vi "RC_Client.vi"(8 "error in (no error)":errorcluster, 10 "ID":i32, 11 "RemoteControl in":refnum<class "RemoteControl.lvclass">) -> (0 "error out":errorcluster)   [LabVIEW 2019, in "RemoteControl.lvlib" / "RemoteControl.lvclass"]
uses:
  RemoteControl.lvclass
  <userlib>/_OpenG.lib/error/error.llb/Filter Error Codes (Array)__ogtk.vi
  b7e1e2dc-a0d6-4bbd-afea-6de24c297ea6.vi
panel:
  in  "milliseconds to wait":u32
  out "time (1 message) (s)":dbl
  out "startup time (s)":dbl
  out "messages/s":dbl
  in  "remote port":u16=6341
  in  "address":string
  out "Response":string
  out "Messages":i32
  in  "Stop":bool
  out "Command reponse":string
  out "Command":string
  out "meta data\n(available commands)":string
  # "CLIENT (API)"
  # "Connection info"
  # "Message Sent"
  # "Message Received"
  # "Metrics"
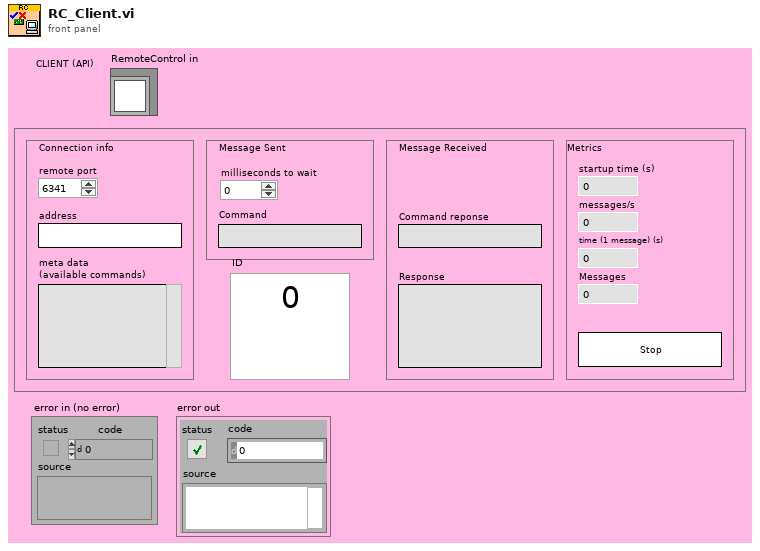
[diagram p1: front panel]
types:
  T1 = cluster{"Command out":string, "Data out":variant, string}
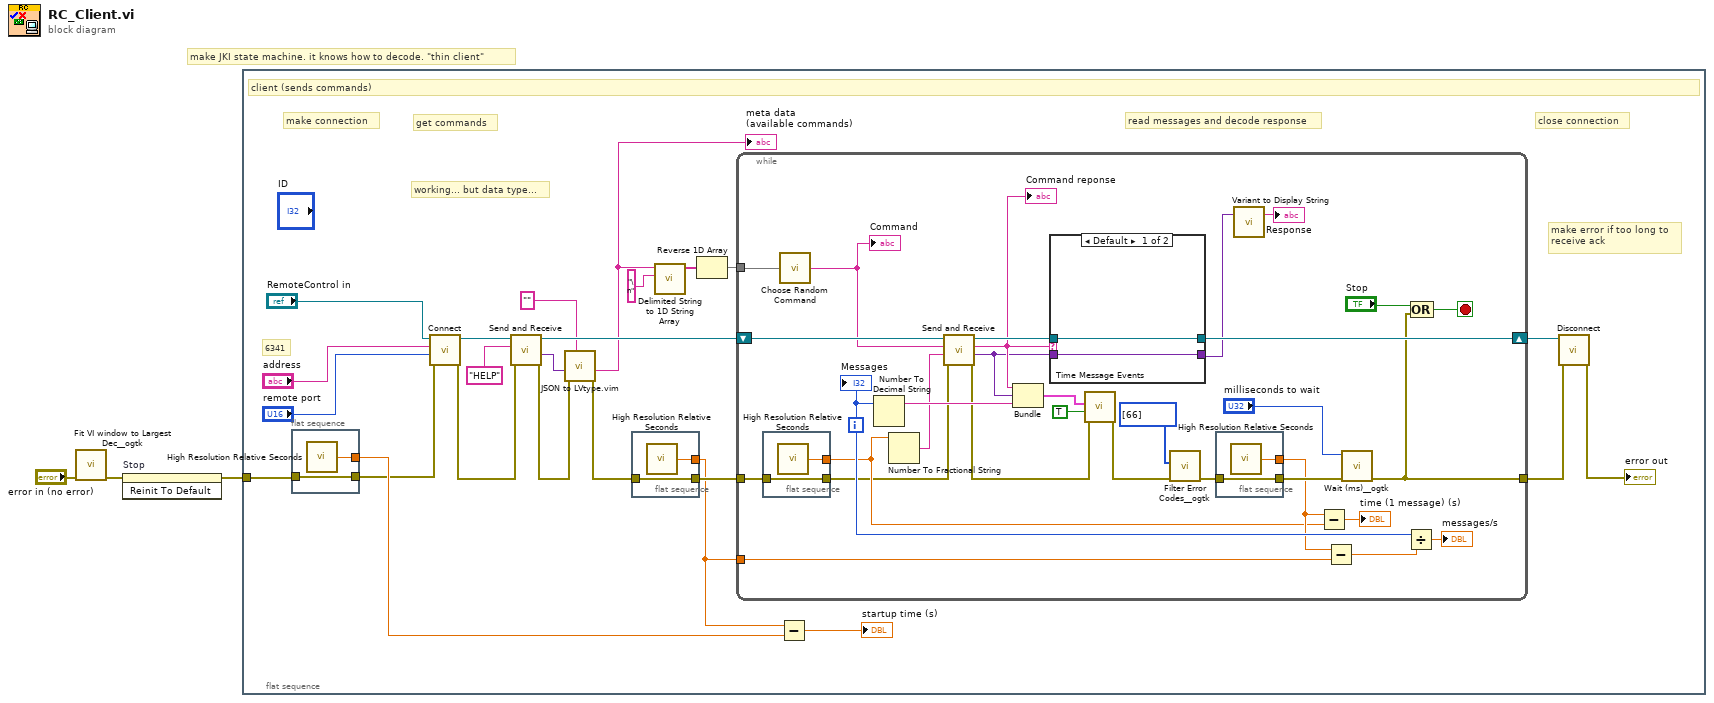
[diagram p0: block diagram]
diagram:
  # "make JKI state machine. it knows how to decode. \"thin client\""
  n1 = call <userlib>:"Fit VI window to Largest Dec__ogtk.vi"("error in (no error)"="error in (no error)") -> ("error out"=w3:errorcluster)  [unwired: 5 in, 1 out]
  n2 = invoke on="Stop" class="Bool" method="Reinit To Default"(error in=w3) -> (error out=w2:errorcluster)  [unwired: 2 in, 2 out]
  n3 = flat-sequence {
    tunnel: w2 -> [w23]
    frame #0 {
      # "working... but data type..."
      # "close connection"
      # "read messages and decode response"
      # "get commands"
      # "make connection"
      # "6341"
      # "make error if too long to\nreceive ack"
      # "client (sends commands)"
      n4 = flat-sequence {
        tunnel: [w28] -> w16
        tunnel: [w29] -> w22
        tunnel: w23 -> [w28]
        frame #0 {
          n5 = call <vilib>:"High Resolution Relative Seconds.vi"() -> ("relative seconds"=w29:dbl)
        }
      }
      n6 = call "Connect.vi"("error in (no error)"=w16, "Port"="remote port", "address"="address", "RemoteControl in"="RemoteControl in") -> ("error out"=w10:errorcluster, "RemoteControl out"=w11:refnum<class "RemoteControl.lvclass">)  [unwired: 6 in]
      n7 = call "Send and Receive.vi"("error in (no error)"=w10, "Command"="HELP", "RemoteControl in"=w11) -> ("error out"=w5:errorcluster, "Data out"=w8:variant, "RemoteControl out"=w9:refnum<class "RemoteControl.lvclass">)  [unwired: 5 in, 1 out]
      n8 = call "JSON to LVtype.vim"("type"="", "error in (no error)"=w5, "JSON Data in"=w8) -> ("error out"=w4:errorcluster, "Data out"=w6:string)  [unwired: 7 in]
      "meta data\n(available commands)" <- w6
      n9 = flat-sequence {
        tunnel: [w30] -> w26
        tunnel: [w31] -> w24
        tunnel: w4 -> [w30]
        frame #0 {
          n10 = call <vilib>:"High Resolution Relative Seconds.vi"() -> ("relative seconds"=w31:dbl)
        }
      }
      n11 = call <vilib>:"Delimited String to 1D String Array.vi"("delimiter"="\n", "delimited string"=w6) -> ("string array"=w21:string[])  [unwired: 9 in]
      n12 = Reverse 1D Array(array=w21) -> (reversed array=w27:string[])
      n13 = while {
        tunnel: [w54] -> w14
        tunnel: w26 -> [w47]
        tunnel: w27 -> [w46]
        tunnel: w24 -> [w57]
        shift-right: [w55] -> w15
        shift-left: w9 -> [w41]
        i -> [w53]
        stop <- w52 stop-if-true
        n14 = flat-sequence {
          tunnel: [w63] -> w38
          tunnel: [w64] -> w44
          tunnel: w47 -> [w63]
          frame #0 {
            n15 = call <vilib>:"High Resolution Relative Seconds.vi"() -> ("relative seconds"=w64:dbl)
          }
        }
        n16 = call "Choose Random Command.vi"("Array"=w46) -> ("String"=w40:string)
        "Command" <- w40
        n17 = Number To Decimal String(number=w53) -> (decimal integer string=w45:string)  [unwired: 1 in]
        n18 = Number To Fractional String(number=w44) -> (F-format string=w39:string)  [unwired: 3 in]
        n19 = call "Send and Receive.vi"("error in (no error)"=w38, "Data"=w39, "Command"=w40, "RemoteControl in"=w41) -> ("error out"=w37:errorcluster, "Data out"=w34:variant, "Command out"=w35:string, "RemoteControl out"=w36:refnum<class "RemoteControl.lvclass">)  [unwired: 4 in]
        "Command reponse" <- w35
        n20 = Bundle("Command out"=w35, "Data out"=w34, w45) -> (w43:T1)  [unwired: 1 in]
        n21 = case shown="Default" w35 {
          tunnel: [w67 w69] -> w32
          tunnel: w36 -> [w68 w70]
          tunnel: w34 -> [w67 w69]
          tunnel: [w68 w70] -> w55
          frame Default {
          }
          frame "HELP" {
          }
        }
        n22 = call "Time Message Events.vi"("error in (no error)"=w37, "Debug Mode"=TRUE, "Message in"=w43) -> ("error out"=w56:errorcluster)  [unwired: 5 in, 3 out]
        n23 = call-poly <userlib>:"Filter Error Codes__ogtk.vi"("Error In"=w56, "Error Codes to Filter"=i32[] [66]) -> ("Error Out"=w51:errorcluster)  [unwired: 7 in, 2 out]
        n24 = flat-sequence {
          tunnel: [w65] -> w50
          tunnel: [w66] -> w49
          tunnel: w51 -> [w65]
          frame #0 {
            n25 = call <vilib>:"High Resolution Relative Seconds.vi"() -> ("relative seconds"=w66:dbl)
          }
        }
        n26 = call "Variant to Display String.vi"("Variant"=w32) -> ("xml string"=→"Response":string)  [unwired: 2 in]
        n27 = Subtract(x=w49, y=w44) -> (x-y=→"time (1 message) (s)":dbl)
        n28 = Subtract(x=w49, y=w57) -> (x-y=w48:dbl)
        n29 = call <userlib>:"Wait (ms)__ogtk.vi"("error in (no error)"=w50, "milliseconds to wait"="milliseconds to wait") -> ("error out"=w54:errorcluster)  [unwired: 8 in, 1 out]
        n30 = Divide(x=w53, y=w48) -> (x/y=→"messages/s":dbl)
        n31 = Compound Arithmetic op=OR("Stop", w54) -> (w52:bool)
        "Messages" <- w53
      }
      n32 = Subtract(x=w24, y=w22) -> (x-y=→"startup time (s)":dbl)
      n33 = call "Disconnect.vi"("error in (no error)"=w14, "RemoteControl in"=w15) -> ("error out"=→"error out":errorcluster)  [unwired: 8 in, 1 out]
    }
  }
